vi "Get Tamer Picture.vi"() -> (0 "Tamer":picture)   [LabVIEW 2020, in "Tamer.lvlib" / "Tamer.lvclass"]
uses:
  Tamer.lvclass
  Tamer.lvclass/Tamer.ctl
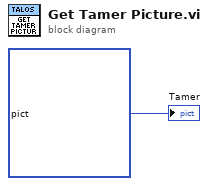
[diagram p0: block diagram]
diagram:
  "Tamer" <- picture bytes[51230] ("Tamer")
